vi "Begin (Christian Colglazier's conflicted copy 2013-02-10).vi"(11 "Image Size":T1=enum."160x120") -> (0 "error out":errorcluster)   [LabVIEW 2012]
doc: "Called before other user functions, this VI is expected to open initial I/O refnums, load in file data, and do all program initialization. Notice that the <B>error out</B> terminal is simply used for data flow. Wiring it to other structures or subVIs ensures that this VI runs first."
uses:
  <vilib>/Rock Robotics/WPI/Camera/WPI_CameraImageSize.ctl
  <vilib>/Rock Robotics/SystemInterfaces/DIO/FPGA_DIOPWMChannel.ctl
  <vilib>/Rock Robotics/WPI/Camera/WPI_CameraWhite Balance Values.ctl
  <vilib>/Rock Robotics/WPI/Camera/WPI_CameraExposure Values.ctl
  <vilib>/Rock Robotics/WPI/Camera/WPI_CameraFrameRate.ctl
  <vilib>/Rock Robotics/WPI/SafetyOutput/WPI_SafetyOutputConfigMenu.ctl
  <vilib>/Rock Robotics/WPI/DriverStation/WPI_DriverStationRobotMode2.ctl
  <vilib>/Rock Robotics/WPI/Joystick/WPI_JoystickDeviceEnum.ctl
  <vilib>/Rock Robotics/SystemInterfaces/DIO/FPGA_DIOChannel.ctl
  <vilib>/Rock Robotics/SystemInterfaces/DIO/FPGA_DIORelayChannel.ctl
  <vilib>/Rock Robotics/WPI/Solenoid/WPI_SolenoidChannel.ctl
  <vilib>/Rock Robotics/SystemInterfaces/AI/FPGA_AIGyroChannel.ctl
  <vilib>/Rock Robotics/SystemInterfaces/AI/FPGA_AIChannel.ctl
  Robot Global Data.vi
  <vilib>/Rock Robotics/WPI/RobotDrive/WPI_RobotDriveOpen4MotorWithJaguar.vi
  <vilib>/Rock Robotics/WPI/MotorControl/WPI_MotorControlOpen Talon.vi
  <vilib>/Rock Robotics/WPI/Solenoid/WPI_SolenoidOpenDouble.vi
  <vilib>/Rock Robotics/WPI/MotorControl/WPI_MotorControlOpen Victor.vi
  <vilib>/Rock Robotics/WPI/Compressor/WPI_CompressorGetSetRefNum.vi
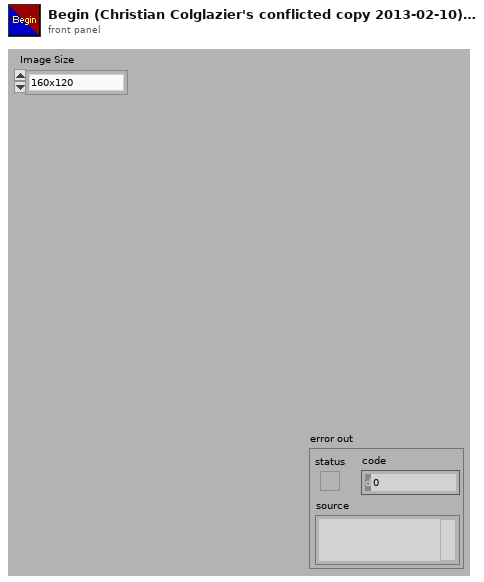
[diagram p1: front panel]
types:
  T1 = typedef "WPI_CameraImageSize.ctl" = enum16{"640x480", "320x240", "160x120"}
  T2 = typedef "FPGA_DIOPWMChannel.ctl" = enum8{"PWM 1", "PWM 2", "PWM 3", "PWM 4", "PWM 5", "PWM 6", "PWM 7", "PWM 8", "PWM 9", "PWM 10", "Invalid"}
  T3 = typedef "FPGA_AIChannel.ctl" = enum8{"AI 1", "AI 2", "AI 3", "AI 4", "AI 5", "AI 6", "AI 7", "AI 8", "Invalid"}
  T4 = typedef "FPGA_AIGyroChannel.ctl" = enum8{"AI 1", "AI 2", "Invalid"}
  T5 = typedef "WPI_SolenoidChannel.ctl" = enum8{"Solenoid 1", "Solenoid 2", "Solenoid 3", "Solenoid 4", "Solenoid 5", "Solenoid 6", "Solenoid 7", "Solenoid 8", "Invalid"}
  T6 = typedef "FPGA_DIORelayChannel.ctl" = enum8{"Relay 1", "Relay 2", "Relay 3", "Relay 4", "Relay 5", "Relay 6", "Relay 7", "Relay 8", "Invalid"}
  T7 = typedef "FPGA_DIOChannel.ctl" = enum8{"DIO 1", "DIO 2", "DIO 3", "DIO 4", "DIO 5", "DIO 6", "DIO 7", "DIO 8", "DIO 9", "DIO 10", "DIO 11", "DIO 12", "DIO 13", "DIO 14", "Invalid"}
  T8 = typedef "WPI_JoystickDeviceEnum.ctl" = enum16{"USB 1", "USB 2", "USB 3", "USB 4", "Kinect 1", "Kinect 2"}
  T9 = typedef "WPI_DriverStationRobotMode2.ctl" = enum16{"Autonomous Disabled", "Autonomous Enabled", "Teleop Disabled", "Teleop Enabled", "Timeout", "Finish", "Test Disabled", "Test Enabled"}
  T10 = typedef "WPI_SafetyOutputConfigMenu.ctl" = enum16{"Enable", "Disable"}
  T11 = typedef "WPI_CameraFrameRate.ctl" = u32
  T12 = typedef "WPI_CameraExposure Values.ctl" = enum16{"Auto", "Flicker-free 50 Hz", "Flicker-free 60 Hz", "Hold current"}
  T13 = typedef "WPI_CameraWhite Balance Values.ctl" = enum16{"Auto", "Fixed indoor", "Fixed outdoor 1", "Fixed outdoor 2", "Fixed fluorescent 1", "Fixed fluorescent 2", "Hold current"}
  T14 = typedef "WPI_MotorControlDeviceRef.ctl" = cluster{"DeviceStatus":errorcluster, "Type":enum16{"PWM", "CAN"}, "PWM":cluster{"Digital Module":T15, "PWM Channel":T2, "DeadBand":T16}, "CAN":cluster{"Device Number":u8, "Control Mode":T17, "Semaphore":T18, "Max Vout":dbl}, "Invert":bool, "TransformRef":T19, "InvTransformRef":T19}
  T15 = typedef "FPGA_TypedefDigitalModule.ctl" = enum16{"Digital Module 1", "Digital Module 2"}
  T16 = typedef "WPI_PWMDeadband.ctl" = cluster{"Name":string, "maxPositivePwm":i32, "minPositivePwm":i32, "centerPwm":i32, "maxNegativePwm":i32, "minNegativePwm":i32, "angularRange":u16}
  T17 = typedef "WPI_CANJaguar_ControlMode.ctl" = enum8{"Percent VBus", "Current", "Speed", "Position", "Voltage"}
  T18 = typedef "Semaphore RefNum" = refnum<k1>
  T19 = typedef "WPI_PWMTransform_ConPane.ctl" = refnum<vi>
  T20 = typedef "WPI_RobotDriveDevRef.ctl" = cluster{"DevStatus":errorcluster, "Motors[]":T14[], "Square Inputs":bool, "Max Output":dbl, "Isochronous":bool}
  T21 = typedef "WPI_CameraDevRef.ctl" = cluster{"Camera Address":string, "CameraStatus":errorcluster, "Acquire Image Notifier":refnum<notifier>}
  T22 = typedef "WPI_JoystickDevRef.ctl" = cluster{"Device":T8}
  T23 = typedef "WPI_SolenoidDevRef.ctl" = cluster{"DevStatus":errorcluster, "Solenoid Module":T24, "Forward Solenoid Channel":T5, "Reverse Solenoid Channel":T5}
  T24 = typedef "FPGA_TypedefSolenoidModule.ctl" = enum16{"Solenoid Module 1", "Solenoid Module 2"}
  T25 = typedef "WPI_GyroDevRef.ctl" = cluster{"DevStatus":errorcluster, "Analog Module":T26, "Analog Channel":T3, "Offset":dbl, "Gain (VoltsPerDegree/Second)":dbl}
  T26 = typedef "FPGA_TypedefAnalogModule.ctl" = enum16{"Analog Module 1", "Analog Module 2"}
  T27 = typedef "WPI_AccelerometerDevRef.ctl" = cluster{"DevStatus":errorcluster, "Analog Module":T26, "Analog Channel":T3, "Scaling":T28}
  T28 = typedef "WPI_AccelerometerScaling.ctl" = cluster{"Gain (VoltsPerG)":dbl, "Center Voltage":dbl}
  T29 = typedef "WPI_CompressorDevRef.ctl" = cluster{"DevStatus":errorcluster, "DigitalInputDevRef":T30, "RelayDevRef":T31}
  T30 = typedef "WPI_DigitalInputDevRef.ctl" = cluster{"DevStatus":errorcluster, "DIO Channel":T7, "Digital Module":T15}
  T31 = typedef "WPI_RelayDevRef.ctl" = cluster{"DevStatus":errorcluster, "Relay Channel":T6, "Digital Module":T15, "Relay Direction":T32}
  T32 = typedef "WPI_RelayDirection.ctl" = enum16{"Both directions", "Forward only", "Reverse only"}
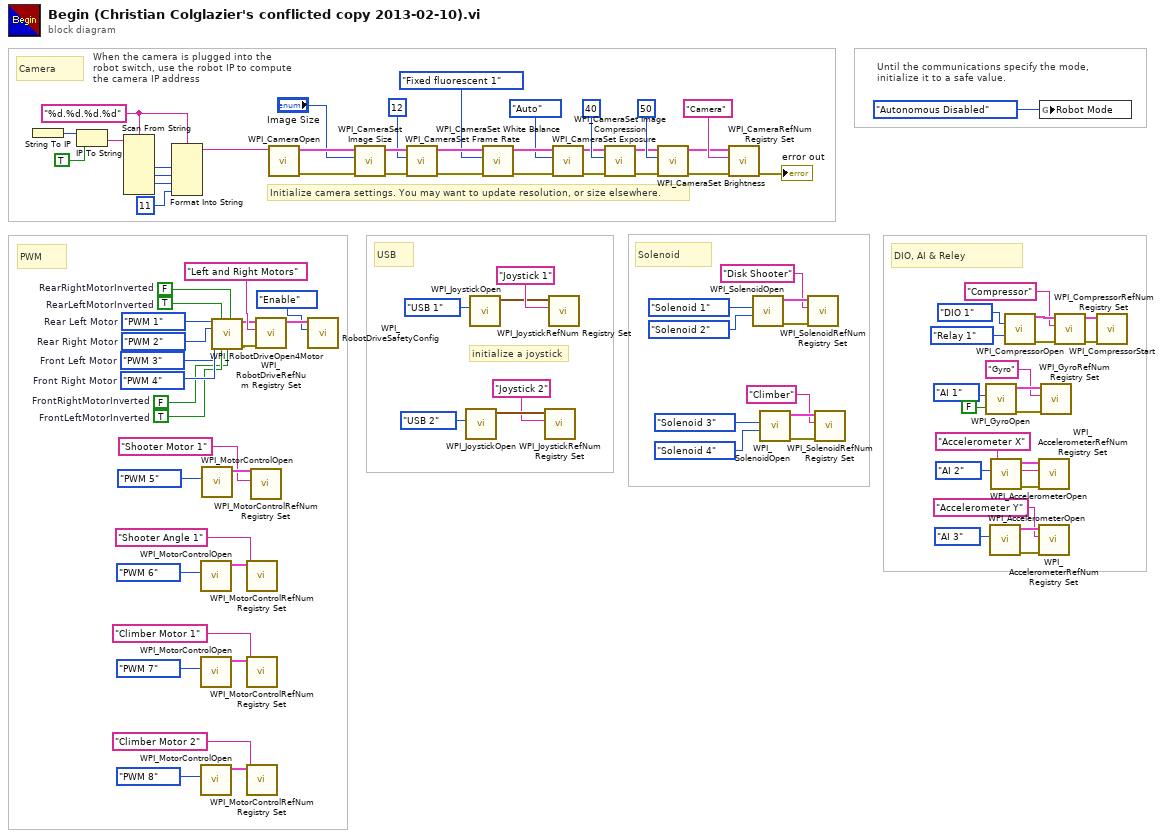
[diagram p0: block diagram]
diagram:
  w47 = TRUE  # FrontLeftMotorInverted
  w46 = FALSE  # FrontRightMotorInverted
  w49 = FPGA_DIOPWMChannel."PWM 4"  # Front Right Motor
  w48 = FPGA_DIOPWMChannel."PWM 3"  # Front Left Motor
  w64 = "%d.%d.%d.%d" ("format string")
  w50 = FPGA_DIOPWMChannel."PWM 2"  # Rear Right Motor
  w51 = FPGA_DIOPWMChannel."PWM 1"  # Rear Left Motor
  w53 = TRUE  # RearLeftMotorInverted
  w52 = FALSE  # RearRightMotorInverted
  # "Camera"
  # "DIO, AI & Reley"
  # "PWM"
  # "Solenoid"
  # "USB"
  # "initialize a joystick"
  # "Until the communications specify the mode,\ninitialize it to a safe value."
  # "When the camera is plugged into the\nrobot switch, use the robot IP to compute\nthe camera IP address"
  # "Initialize camera settings. You may want to update resolution, or size elsewhere."
  n1 = String To IP() -> (0:w71:u32)  [unwired: 1 in]
  n2 = IP To String(1:TRUE ("dot notation? (F)"), 2:w71) -> (0:w69:string)
  n3 = Scan From String(format string=w64, input string=w69) -> (output 1=w68:i32, output 2=w67:i32, output 3=w66:i32)  [unwired: 7 in, 3 out]
  n4 = Format Into String(format string=w64, w68, w67, w66, 11 ("Compression")) -> (resulting string=w60:string)  [unwired: 2 in, 1 out]
  n5 = call-poly <vilib>:"WPI_MotorControlOpen.vi"("PWM Channel"=FPGA_DIOPWMChannel."PWM 6") -> ("MotorControlDeviceRef"=w41:T14)  [unwired: 9 in, 1 out]
  n6 = call-poly <vilib>:"WPI_MotorControlOpen.vi"("PWM Channel"=FPGA_DIOPWMChannel."PWM 7") -> ("MotorControlDeviceRef"=w5:T14)  [unwired: 9 in, 1 out]
  n7 = call-poly <vilib>:"WPI_MotorControlOpen.vi"("PWM Channel"=FPGA_DIOPWMChannel."PWM 8") -> ("MotorControlDeviceRef"=w2:T14)  [unwired: 9 in, 1 out]
  n8 = call-poly <vilib>:"WPI_MotorControlOpen.vi"("PWM Channel"=FPGA_DIOPWMChannel."PWM 5") -> ("MotorControlDeviceRef"=w44:T14)  [unwired: 9 in, 1 out]
  n9 = call-poly <vilib>:"WPI_RobotDriveOpen4Motor.vi"("Rear Left Motor"=w51, "Rear Left Motor Inverted"=w53, "Rear Right Motor Inverted"=w52, "Rear Right Motor"=w50, "Front Left Motor"=w48, "Front Right Motor"=w49, "Front Left Motor Inverted"=w47, "Front Right Motor Inverted"=w46) -> ("RobotDriveDevRef"=w54:T20, "error out"=w55:errorcluster)  [unwired: 6 in]
  n10 = call <vilib>:"WPI_MotorControlRefNum Registry Set.vi"("refnum name"="Shooter Angle 1", "MotorControlDevRef"=w41) -> ()  [unwired: 8 in, 2 out]
  n11 = call <vilib>:"WPI_MotorControlRefNum Registry Set.vi"("refnum name"="Climber Motor 1", "MotorControlDevRef"=w5) -> ()  [unwired: 8 in, 2 out]
  n12 = call <vilib>:"WPI_MotorControlRefNum Registry Set.vi"("refnum name"="Climber Motor 2", "MotorControlDevRef"=w2) -> ()  [unwired: 8 in, 2 out]
  n13 = call <vilib>:"WPI_MotorControlRefNum Registry Set.vi"("refnum name"="Shooter Motor 1", "MotorControlDevRef"=w44) -> ()  [unwired: 8 in, 2 out]
  n14 = call <vilib>:"WPI_RobotDriveRefNum Registry Set.vi"("error in (no error)"=w55, "refnum name"="Left and Right Motors", "RobotDriveDevRef"=w54) -> ("RobotDriveDevRef"=w63:T20)  [unwired: 8 out]
  n15 = call <vilib>:"WPI_CameraOpen.vi"("Camera Address"=w60) -> ("error out"=w83:errorcluster, "CameraDevRef"=w84:T21)  [unwired: 1 in, 8 out]
  n16 = call <vilib>:"WPI_RobotDriveSafetyConfig.vi"("mode"=WPI_SafetyOutputConfigMenu."Enable", "RobotDriveDevRef"=w63) -> ()  [unwired: 8 in, 2 out]
  n17 = call <vilib>:"WPI_CameraSet Image Size.vi"("error in (no error)"=w83, "Image Size"="Image Size", "CameraDevRef"=w84) -> ("error out"=w82:errorcluster, "CameraDevRef Out"=w85:T21)  [unwired: 7 out]
  n18 = call <vilib>:"WPI_CameraSet Frame Rate.vi"("error in (no error)"=w82, "Frame Rate (fps)"=T11 12, "CameraDevRef"=w85) -> ("error out"=w81:errorcluster, "CameraDevRef Out"=w87:T21)  [unwired: 7 out]
  n19 = call <vilib>:"WPI_JoystickOpen.vi"("JoystickDevice"=WPI_JoystickDeviceEnum."USB 2") -> ("JoystickDevRef"=w38:T22)  [unwired: 10 in]
  n20 = call <vilib>:"WPI_JoystickOpen.vi"("JoystickDevice"=WPI_JoystickDeviceEnum."USB 1") -> ("JoystickDevRef"=w58:T22)  [unwired: 10 in]
  n21 = call <vilib>:"WPI_CameraSet White Balance.vi"("error in (no error)"=w81, "White Balance"=WPI_CameraWhite_Balance_Values."Fixed fluorescent 1", "CameraDevRef"=w87) -> ("error out"=w80:errorcluster, "CameraDevRef Out"=w86:T21)  [unwired: 7 out]
  n22 = call <vilib>:"WPI_JoystickRefNum Registry Set.vi"("refnum name"="Joystick 2", "JoystickDevRef"=w38) -> ()  [unwired: 8 in, 2 out]
  n23 = call <vilib>:"WPI_JoystickRefNum Registry Set.vi"("refnum name"="Joystick 1", "JoystickDevRef"=w58) -> ()  [unwired: 8 in, 2 out]
  n24 = call <vilib>:"WPI_CameraSet Exposure.vi"("error in (no error)"=w80, "Exposure"=WPI_CameraExposure_Values."Auto", "CameraDevRef"=w86) -> ("error out"=w79:errorcluster, "CameraDevRef Out"=w89:T21)  [unwired: 7 out]
  n25 = call <vilib>:"WPI_CameraSet Image Compression.vi"("error in (no error)"=w79, "Compression"=40, "CameraDevRef"=w89) -> ("error out"=w78:errorcluster, "CameraDevRef Out"=w88:T21)  [unwired: 7 out]
  n26 = call <vilib>:"WPI_CameraSet Brightness.vi"("error in (no error)"=w78, "Brightness"=50, "CameraDevRef"=w88) -> ("error out"=w76:errorcluster, "CameraDevRef Out"=w77:T21)  [unwired: 7 out]
  n27 = call <vilib>:"WPI_CameraRefNum Registry Set.vi"("error in (no error)"=w76, "refnum name"="Camera", "CameraDevRef"=w77) -> ("error out"=→"error out":errorcluster)  [unwired: 8 out]
  n28 = call-poly <vilib>:"WPI_SolenoidOpen.vi"("Reverse Solenoid Channel"=WPI_SolenoidChannel."Solenoid 2" ("Forward Solenoid Channel"), "Forward Solenoid Channel"=WPI_SolenoidChannel."Solenoid 1" ("Solenoid Channel")) -> ("error out"=w28:errorcluster, "SolenoidDevRef"=w27:T23)  [unwired: 8 in]
  n29 = call-poly <vilib>:"WPI_SolenoidOpen.vi"("Reverse Solenoid Channel"=WPI_SolenoidChannel."Solenoid 4" ("Forward Solenoid Channel"), "Forward Solenoid Channel"=WPI_SolenoidChannel."Solenoid 3" ("Solenoid Channel")) -> ("error out"=w23:errorcluster, "SolenoidDevRef"=w24:T23)  [unwired: 8 in]
  n30 = call <vilib>:"WPI_SolenoidRefNum Registry Set.vi"("error in (no error)"=w28, "refnum name"="Disk Shooter", "SolenoidDevRef"=w27) -> ()  [unwired: 7 in, 2 out]
  n31 = call <vilib>:"WPI_SolenoidRefNum Registry Set.vi"("error in (no error)"=w23, "refnum name"="Climber", "SolenoidDevRef"=w24) -> ()  [unwired: 7 in, 2 out]
  n32 = call <vilib>:"WPI_GyroOpen.vi"("Calibrate On Open"=FALSE, "Analog Channel"=FPGA_AIGyroChannel."AI 1") -> ("error out"=w19:errorcluster, "GyroDevRef"=w18:T25)  [unwired: 7 in, 1 out]
  n33 = call <vilib>:"WPI_AccelerometerOpen.vi"("Analog Channel"=FPGA_AIChannel."AI 3") -> ("error out"=w9:errorcluster, "AccelerometerDevRef"=w8:T27)  [unwired: 3 in, 6 out]
  n34 = call <vilib>:"WPI_AccelerometerOpen.vi"("Analog Channel"=FPGA_AIChannel."AI 2") -> ("error out"=w12:errorcluster, "AccelerometerDevRef"=w11:T27)  [unwired: 3 in, 6 out]
  n35 = call <vilib>:"WPI_CompressorOpen.vi"("Pressure Switch DIO Channel"=FPGA_DIOChannel."DIO 1", "Relay Channel"=FPGA_DIORelayChannel."Relay 1") -> ("CompressorDevRef"=w34:T29, "error out"=w31:errorcluster)  [unwired: 12 in]
  n36 = call <vilib>:"WPI_AccelerometerRefNum Registry Set.vi"("error in (no error)"=w12, "refnum name"="Accelerometer X", "AccelerometerDevRef"=w11) -> ()  [unwired: 7 in, 2 out]
  n37 = call <vilib>:"WPI_AccelerometerRefNum Registry Set.vi"("error in (no error)"=w9, "refnum name"="Accelerometer Y", "AccelerometerDevRef"=w8) -> ()  [unwired: 7 in, 2 out]
  n38 = global write "Robot Global Data.vi" "Robot Mode"(WPI_DriverStationRobotMode2."Autonomous Disabled" ("Robot Mode")) -> ()
  n39 = call <vilib>:"WPI_GyroRefNum Registry Set.vi"("error in (no error)"=w19, "refnum name"="Gyro", "GyroDevRef"=w18) -> ()  [unwired: 7 in, 2 out]
  n40 = call <vilib>:"WPI_CompressorRefNum Registry Set.vi"("error in (no error)"=w31, "refnum name"="Compressor", "CompressorDevRef"=w34) -> ("error out"=w36:errorcluster, "CompressorDevRef"=w35:T29)  [unwired: 7 in]
  n41 = call <vilib>:"WPI_CompressorStart.vi"("error in (no error)"=w36, "CompressorDevRef"=w35) -> ()  [unwired: 8 in, 2 out]
